vi "Find Responce Body Parameter.vi"(10 "Body Parameters in":T1[](array[typedef]), 11 "Parameter name":string) -> (2 "Body Parameter":T1, 3 "Found?":bool)   [LabVIEW 2017]
uses:
  Types/Body Parameter Type.ctl
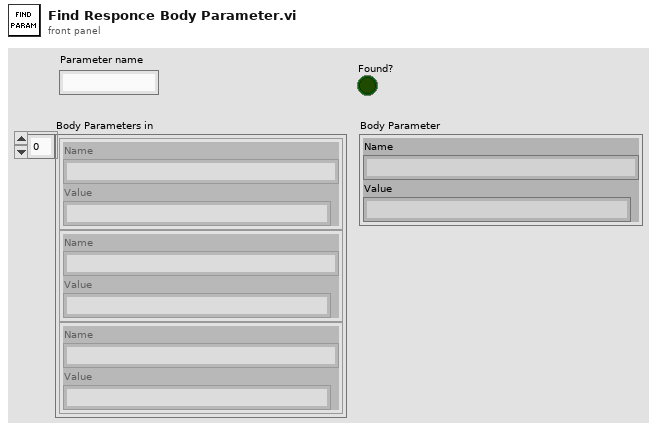
[diagram p1: front panel]
types:
  T1 = typedef "Body Parameter Type.ctl" = cluster{"Name":string, "Value":string}
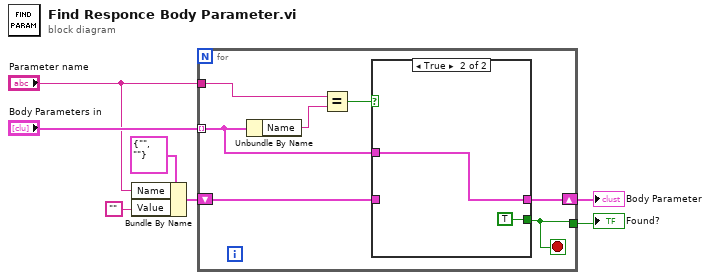
[diagram p0: block diagram]
diagram:
  n1 = Bundle By Name(cluster=T1 {"Name"="", "Value"=""} ("Body Parameter"), "Name"="Parameter name", "Value"="") -> (w3:T1)
  n2 = for {
    tunnel: "Body Parameters in" -> [w10] mode=indexing
    tunnel: "Parameter name" -> [w14]
    shift-right: [w11] -> w2
    shift-left: w3 -> [w9]
    tunnel: [w8] -> w1
    stop <- w8 stop-if-true
    n3 = Unbundle By Name(w10) -> ("Name"=w13:string)
    n4 = Equal?(x=w14, y=w13) -> (x = y?=w12:bool)
    n5 = case shown="True" w12 {
      tunnel: [w15 w17] -> w11
      tunnel: w10 -> [_ w17]
      tunnel: w9 -> [w15 _]
      tunnel: [_ TRUE] -> w8
      frame False {
      }
      frame True {
      }
    }
  }
  "Body Parameter" <- w2
  "Found?" <- w1
